vi "Shutdown_Criteria_HGB2.vi"(8 "error in (no error)":errorcluster, 9 "Dummy Variable 2":dbl=1.0, 11 "Data Array":dbl[](array[numeric])) -> (0 "error out":errorcluster, 3 "Enum":T1=enum."Shutdown")   [LabVIEW 2016]
uses:
  Producer_Case_Structure.ctl
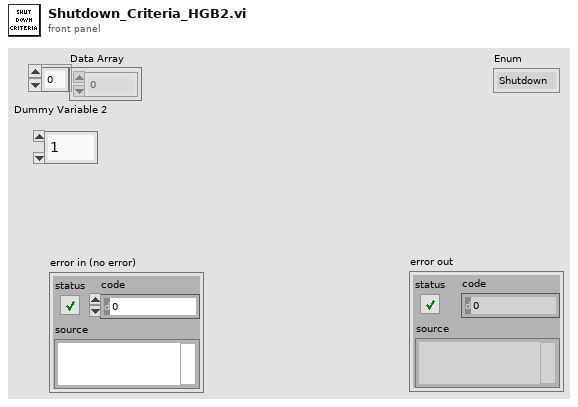
[diagram p1: front panel]
types:
  T1 = typedef "Producer_Case_Structure.ctl" = enum16{"Initialize", "Read", "Write", "Display", "Queue", "Evaluate", "Error", "Shutdown"}
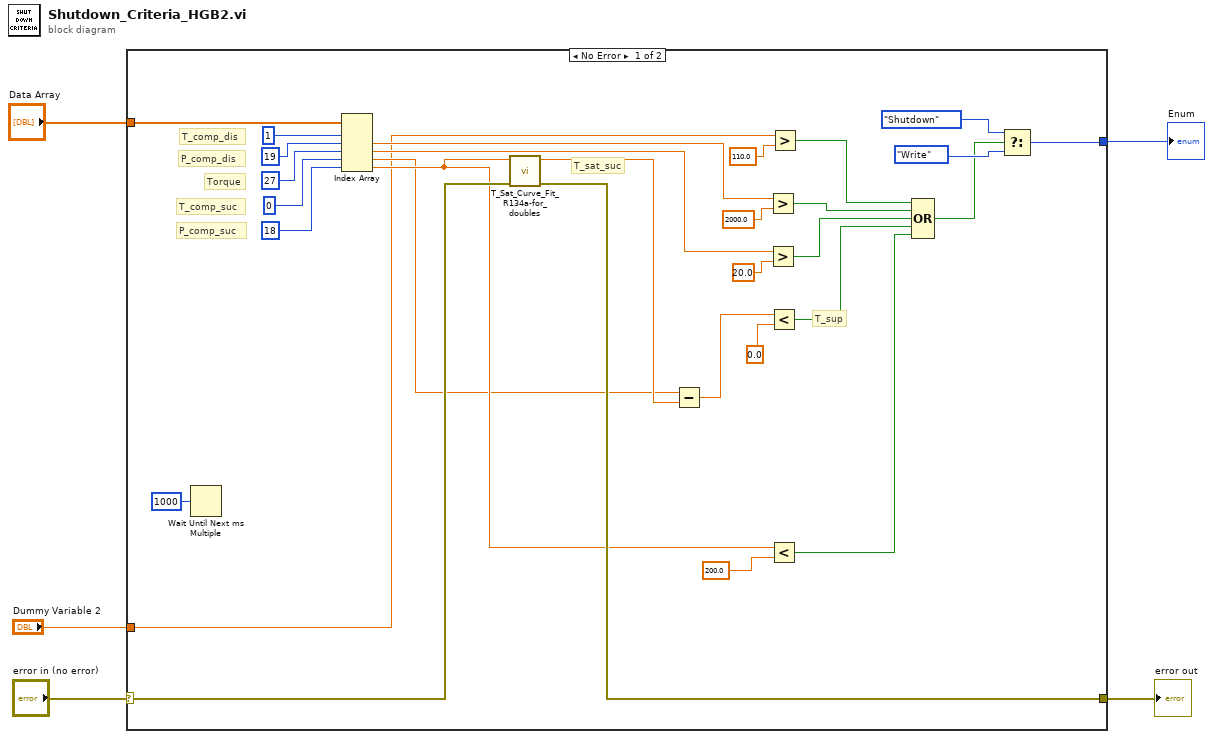
[diagram p0: block diagram]
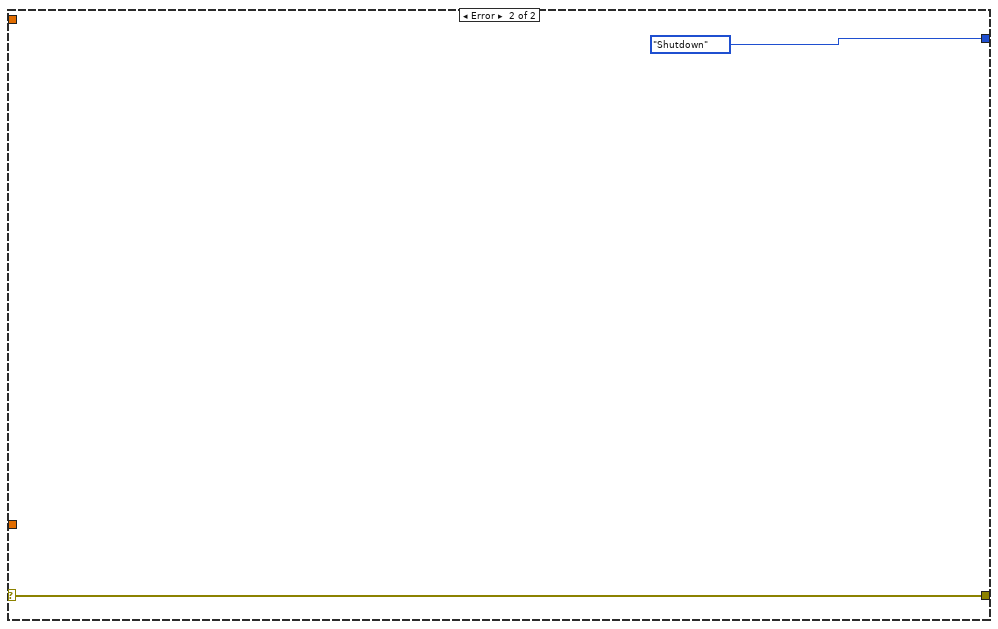
[diagram p2: hidden frame]
diagram:
  n1 = case shown="No Error" "error in (no error)" {
    selector: "error in (no error)" -> [w14 w37]
    tunnel: "Data Array" -> [w33 _]
    tunnel: [w13 w37] -> w3
    tunnel: "Dummy Variable 2" -> [w6 _]
    tunnel: [w30 Producer_Case_Structure."Shutdown" ("Enum")] -> w1
    frame No Error {
      # "T_sup"
      # "T_sat_suc"
      # "P_comp_suc"
      # "T_comp_suc"
      # "Torque"
      # "P_comp_dis"
      # "T_comp_dis"
      n2 = Wait Until Next ms Multiple(millisecond multiple=u32 1000) -> ()  [unwired: 1 out]
      n3 = Index Array(array=w33, index #1=1 ("index"), index #2=19 ("index"), index #3=27 ("index"), index #4=0 ("index"), index #5=18 ("index")) -> (element #2=w24:dbl, element #3=w20:dbl, element #4=w10:dbl, element #5=w12:dbl)  [unwired: 1 out]
      n4 = call "T_Sat_Curve_Fit_R134a-for_doubles.vi"("error in (no error)"=w14, "Numeric in"=w12) -> ("error out"=w13:errorcluster, "Numeric out"=w11:dbl)  [unwired: 8 in]
      n5 = Subtract(x=w10, y=w11) -> (x-y=w9:dbl)
      n6 = Greater?(x=w24, y=2000.0) -> (0:w23:bool)
      n7 = Greater?(x=w20, y=20.0) -> (0:w19:bool)
      n8 = Less?(x=w9, y=0.0) -> (x < y?=w16:bool)
      n9 = Less?(x=w12, y=200.0) -> (x < y?=w15:bool)
      n10 = Greater?(x=w6, y=110.0) -> (0:w7:bool)
      n11 = Compound Arithmetic op=OR(w7, w23, w19, w16, w15) -> (w22:bool)
      n12 = Select(t=Producer_Case_Structure."Shutdown" ("Enum"), s=w22, f=Producer_Case_Structure."Write" ("Enum")) -> (s? t:f=w30:T1)
    }
    frame Error {
    }
  }
  "error out" <- w3
  "Enum" <- w1
